vi "Auto Gyro Go To Zero.vi"(11 "Run?":bool) -> (3 "Done":bool)   [LabVIEW 2013]
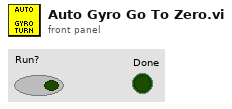
[diagram p1: front panel]
types:
  T1 = typedef "WPI_I2CDevRef.ctl" = cluster{"DevStatus":errorcluster, "Digital Module":T2, "Device Address":u8}
  T2 = typedef "FPGA_TypedefDigitalModule.ctl" = enum16{"Digital Module 1", "Digital Module 2"}
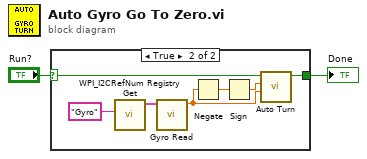
[diagram p0: block diagram]
diagram:
  n1 = case shown="True" "Run?" {
    selector: "Run?" -> [w3 w8]
    tunnel: [w3 w7] -> w1
    frame False {
    }
    frame True {
      n2 = call <vilib>:"WPI_I2CRefNum Registry Get.vi"("refnum name"="Gyro") -> ("I2CDevRef"=w10:T1)  [unwired: 9 in, 1 out]
      n3 = call "Gyro Read.vi"("I2CDevRef In"=w10) -> ("Angle"=w4:dbl)  [unwired: 9 in, 1 out]
      n4 = Negate(x=w4) -> (-x=w6:dbl)
      n5 = Sign(1:w6) -> (0:w5:dbl)
      n6 = call "Auto Turn.vi"("Turn Amount"=w4, "+/-?"=w5, "Run?"=w8) -> ("Done"=w7:bool)  [unwired: 8 in]
    }
  }
  "Done" <- w1
